vi "Convert Result Units.vi"(8 "error in (no error)":errorcluster, 9 "Convert to unit":T1, 10 "Result in":dbl[](array[numeric]), 11 "Keithley 622x2182 Driver in":refnum<class "Keithley 622x2182 Driver.lvclass">) -> (0 "error out":errorcluster, 2 "Result out":dbl[](array[numeric]), 3 "Keithley 622x2182 Driver out":refnum<class "Keithley 622x2182 Driver.lvclass">)   [LabVIEW 2021, in "Keithley 622x2182 Driver.lvclass"]
uses:
  Keithley 622x2182 Driver.lvclass
  Unit.ctl
  Keithley 622x2182 Driver.lvclass/Keithley 622x2182 Driver.ctl
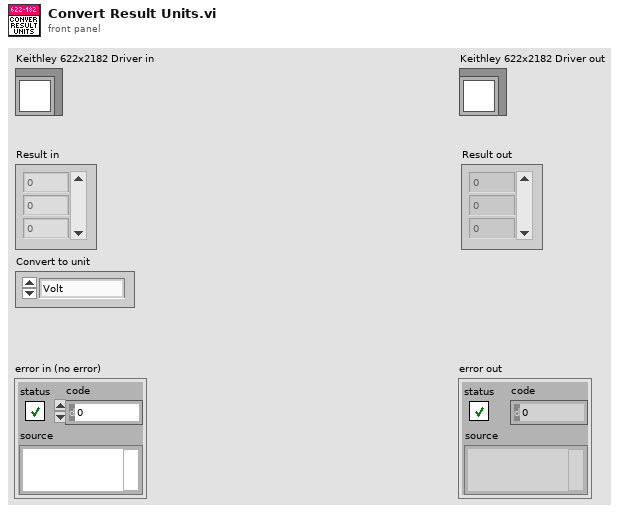
[diagram p1: front panel]
types:
  T1 = typedef "Unit.ctl" = enum16{"Volt", "Ohm", "Siemens"}
  T2 = typedef "Stepper Config.ctl" = cluster{"Start":dbl, "End":dbl, "Step":dbl, "Delta":dbl, "Scan shape":enum16{"Sawtooth", "Triangular"}, "Append measurements":string[], "Pulse width":dbl, "Pulse interval":dbl, "Scan mode":enum16{"Delta", "Diff. conductance", "Pulse delta sweep"}}
  T3 = enum16{"Delta", "Diff. conductance", "Pulse delta sweep"}
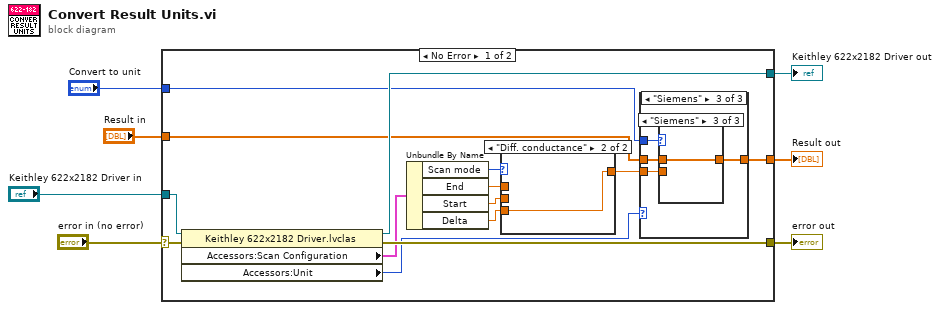
[diagram p0: block diagram]
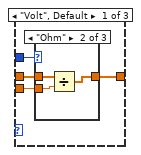
[diagram p2: hidden frame]
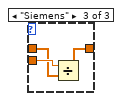
[diagram p4: hidden frame]
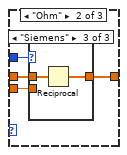
[diagram p5: hidden frame]
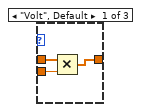
[diagram p6: hidden frame]
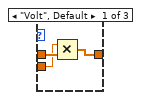
[diagram p8: hidden frame]
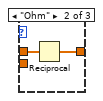
[diagram p9: hidden frame]
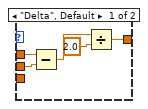
[diagram p10: hidden frame]
diagram:
  n1 = case shown="No Error" "error in (no error)" {
    selector: "error in (no error)" -> [w21 w61]
    tunnel: [w20 w61] -> w6
    tunnel: [w18 w60] -> w4
    tunnel: "Keithley 622x2182 Driver in" -> [w19 w60]
    tunnel: "Convert to unit" -> [w12 _]
    tunnel: "Result in" -> [w11 w59]
    tunnel: [w10 w59] -> w1
    frame No Error {
      n2 = property class="Keithley 622x2182 Driver.lvclas"(reference=w19, error in=w21) -> (reference out=w18:refnum<class "Keithley 622x2182 Driver.lvclass">, error out=w20:errorcluster, "Accessors:Scan Configuration"=w17:T2, "Accessors:Unit"=w13:T1)
      n3 = Unbundle By Name(w17) -> ("Scan mode"=w16:T3, "End"=w15:dbl, "Start"=w14:dbl, "Delta"=w8:dbl)
      n4 = case shown="\"Diff. conductance\"" w16 {
        tunnel: w15 -> [w57 _]
        tunnel: w14 -> [w56 _]
        tunnel: [w54 w58] -> w9
        tunnel: w8 -> [_ w58]
        frame "Delta", Default {
          n5 = Subtract(x=w57, y=w56) -> (x-y=w55:dbl)
          n6 = Divide(x=w55, y=2.0) -> (x/y=w54:dbl)
        }
        frame "Diff. conductance" {
        }
      }
      n7 = case shown="\"Siemens\"" w13 {
        tunnel: w12 -> [w22 w36 w46]
        tunnel: w11 -> [w25 w35 w45]
        tunnel: [w24 w34 w44] -> w10
        tunnel: w9 -> [w23 w33 w43]
        frame "Volt", Default {
          n8 = case shown="\"Ohm\"" w22 {
            tunnel: w25 -> [w26 w29 w31]
            tunnel: [w26 w27 w30] -> w24
            tunnel: w23 -> [_ w28 w32]
            frame "Volt", Default {
            }
            frame "Ohm" {
              n9 = Divide(x=w29, y=w28) -> (x/y=w27:dbl[])
            }
            frame "Siemens" {
              n10 = Divide(x=w32, y=w31) -> (x/y=w30:dbl[])
            }
          }
        }
        frame "Ohm" {
          n11 = case shown="\"Siemens\"" w36 {
            tunnel: w35 -> [w39 w40 w42]
            tunnel: [w38 w40 w41] -> w34
            tunnel: w33 -> [w37 _ _]
            frame "Volt", Default {
              n12 = Multiply(x=w39, y=w37) -> (x*y=w38:dbl[])
            }
            frame "Ohm" {
            }
            frame "Siemens" {
              n13 = Reciprocal(x=w42) -> (1/x=w41:dbl[])
            }
          }
        }
        frame "Siemens" {
          n14 = case shown="\"Siemens\"" w46 {
            tunnel: w45 -> [w48 w51 w52]
            tunnel: [w49 w50 w52] -> w44
            tunnel: w43 -> [w47 _ _]
            frame "Volt", Default {
              n15 = Multiply(x=w47, y=w48) -> (x*y=w49:dbl[])
            }
            frame "Ohm" {
              n16 = Reciprocal(x=w51) -> (1/x=w50:dbl[])
            }
            frame "Siemens" {
            }
          }
        }
      }
    }
    frame Error {
    }
  }
  "error out" <- w6
  "Keithley 622x2182 Driver out" <- w4
  "Result out" <- w1
